vi "Dsc_BoardElecMan.vi"(8 "error in":errorcluster) -> (0 "error out":errorcluster)   [LabVIEW 2014, in "DscBoardDistributeElectrodes.lvlib"]
uses:
  DscBoardDistributeElectrodes.lvlib
  <vilib>/Utility/miscctls.llb/LVRowAndColumnTypeDef.ctl
  DataBase/DataBase.lvlib
  DetectElecrodes/DetectElectros.lvlib
panel:
  out "元素":string
  in  "全部移除":bool
  in  "移除":bool
  in  "采集卡列表":u16(ring) items=["2号数据采集板", "3号数据采集板", "4号数据采集板", "5号数据采集版", "6号数据采集板", "7号数据采集板", "8号数据采集板", "9号数据采集板", "10号数据采集板", "11号数据采集板", "12号数据采集板", "13号数据采集板", "14号数据采集板", "1号数据采集板"]
  in  "已配置 采集卡-检测电极":i32(listbox)
  in  "添加":bool
  in  "电极编号":i32(listbox)
  in  "未配置 采集卡-检测电极":i32(listbox)
  in  "区域":u16(ring)
  in  "退出":bool
  in  "OK":bool
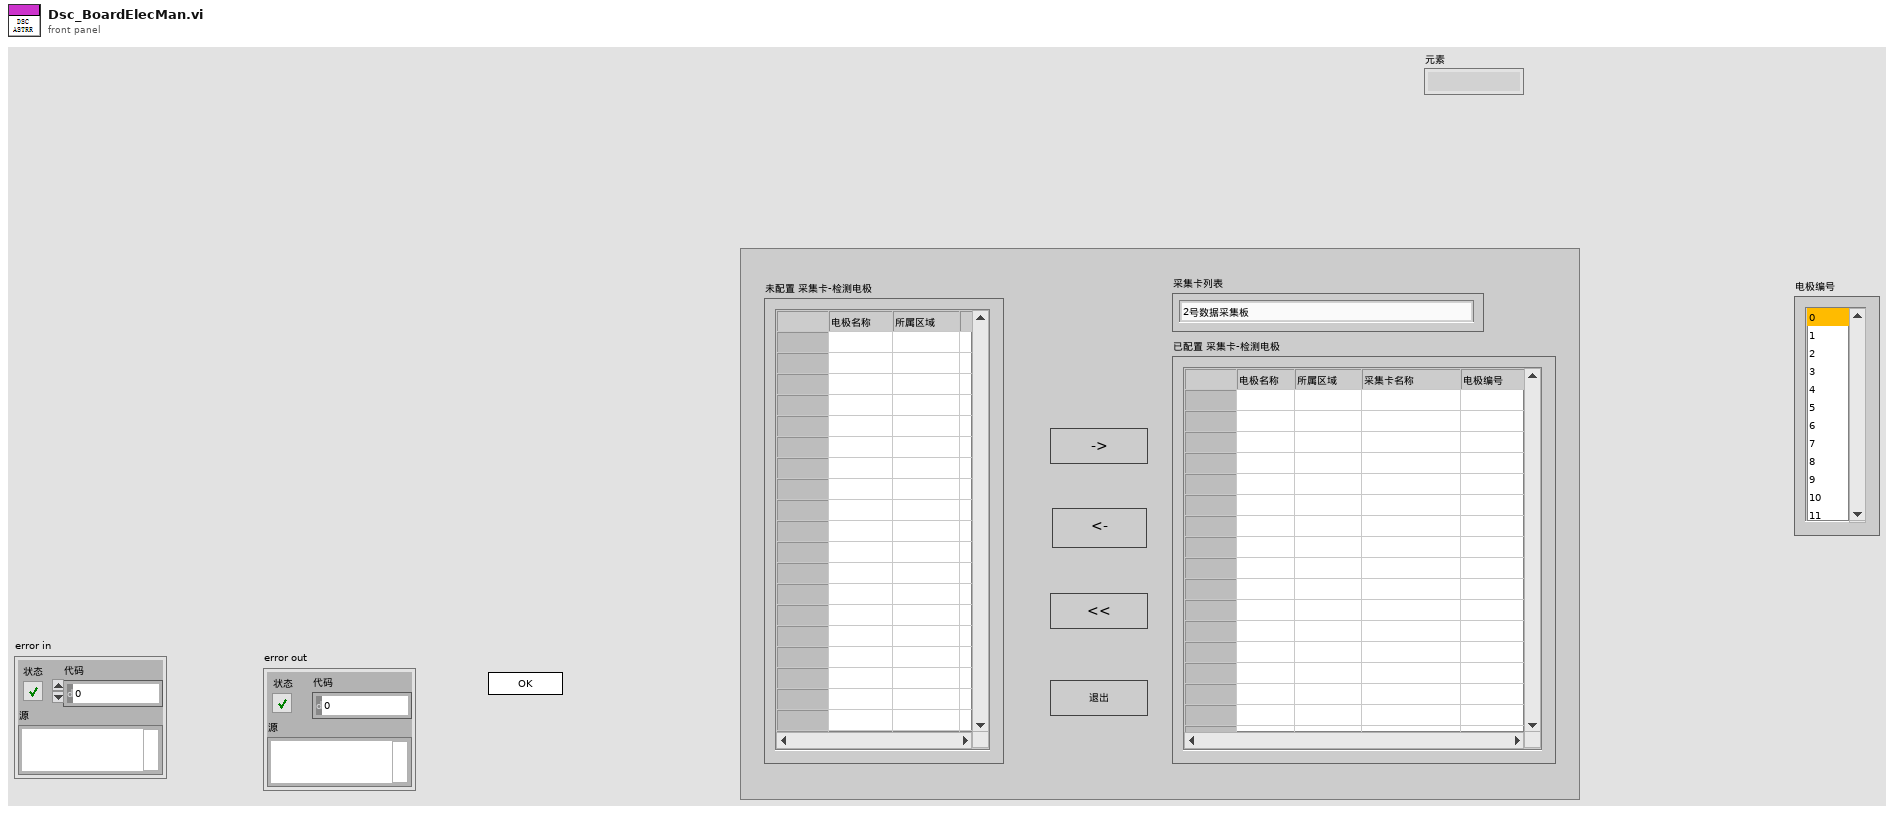
[diagram p1: front panel]
types:
  T1 = enum32{"invalid app kind", "Development System", "Run Time System", "Student Edition", "Embedded LabVIEW", "Evaluation", "Custom"}
  T2 = enum32{"Invalid", "Standard", "Closed", "Hidden", "Minimized", "Maximized"}
  T3 = typedef "LVRowAndColumnTypeDef.ctl" = cluster{"Row":i32, "Column":i32}
  T4 = cluster{"Core":cluster{"Current VI Reference":refnum<vi>, "Close Panel on Exit?":bool}, "Your Boolean data":bool, "Your string data":string, "未配置Dsc行列":T3, "DscInfo":cluster{"DscName":string, "DscAddress":string}, "Dsc":string[][], "Dsc列表":i32, "已配置Dsc行列":T3, "Dsc板名称":string}
  T5 = typedef "LVPoint32TypeDef.ctl" = cluster{"Horizontal":i32, "Vertical":i32}
  T6 = cluster{"Current VI Reference":refnum<vi>, "Close Panel on Exit?":bool}
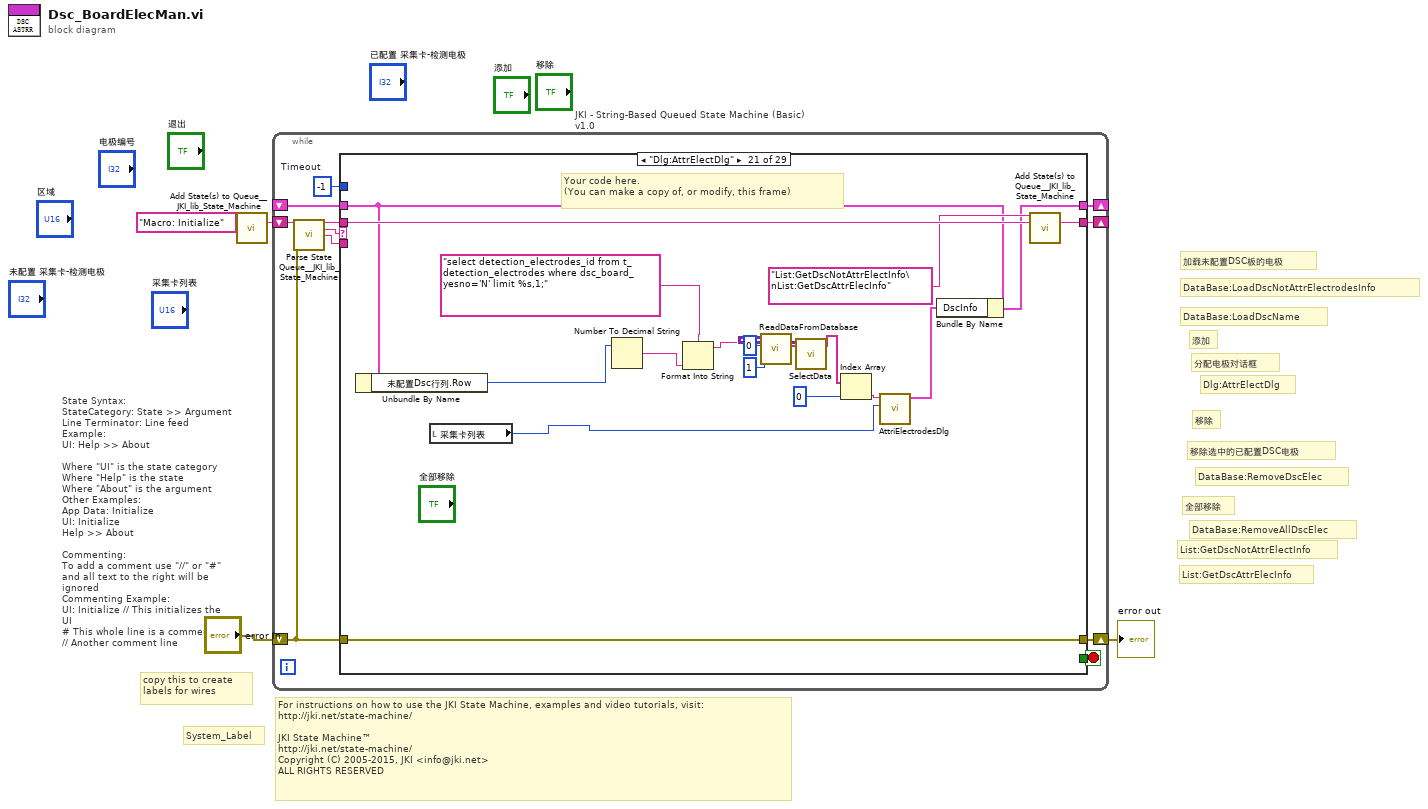
[diagram p0: block diagram]
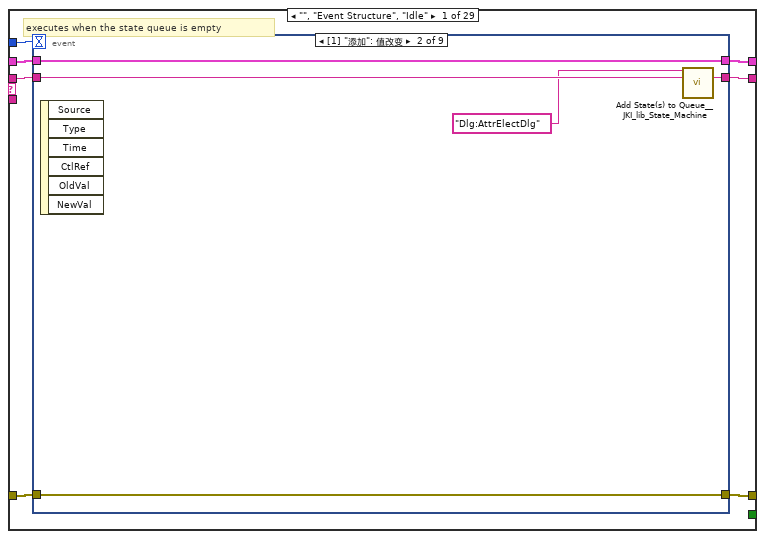
[diagram p2: hidden frame]
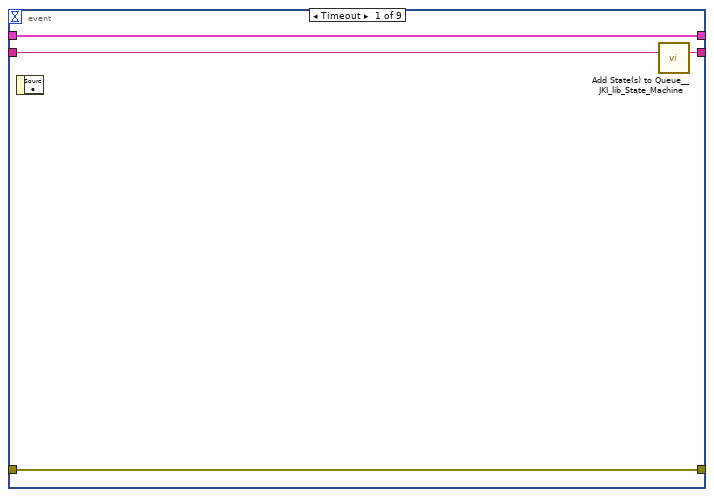
[diagram p3: hidden frame]
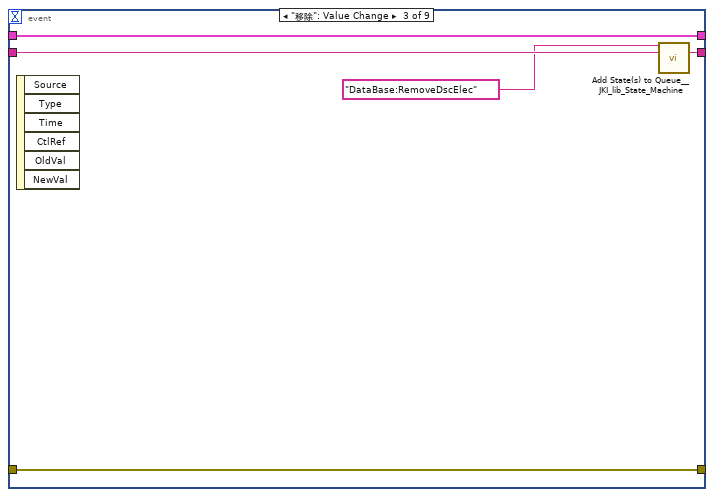
[diagram p4: hidden frame]
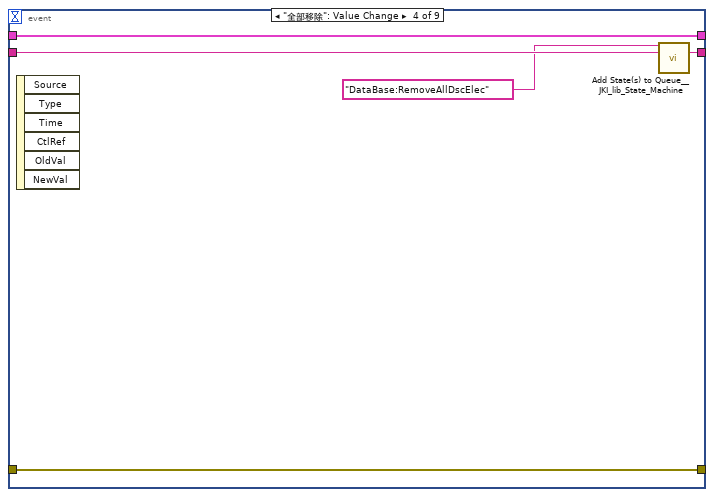
[diagram p5: hidden frame]
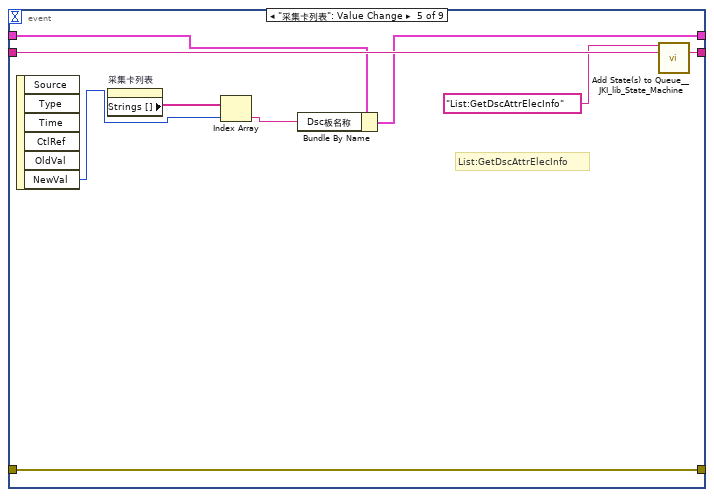
[diagram p6: hidden frame]
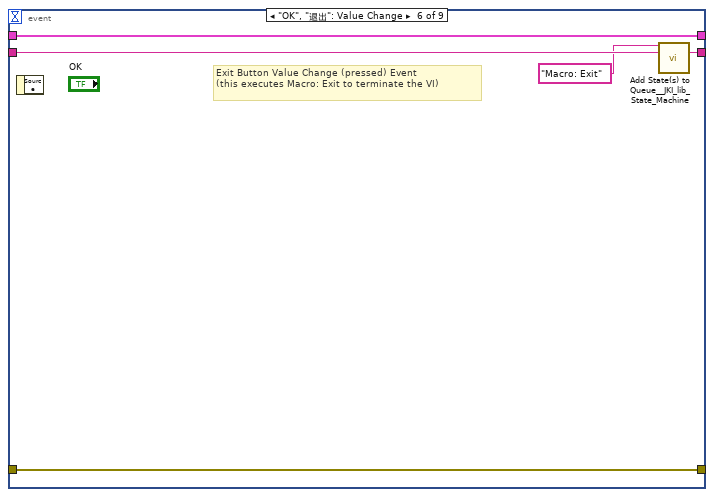
[diagram p7: hidden frame]
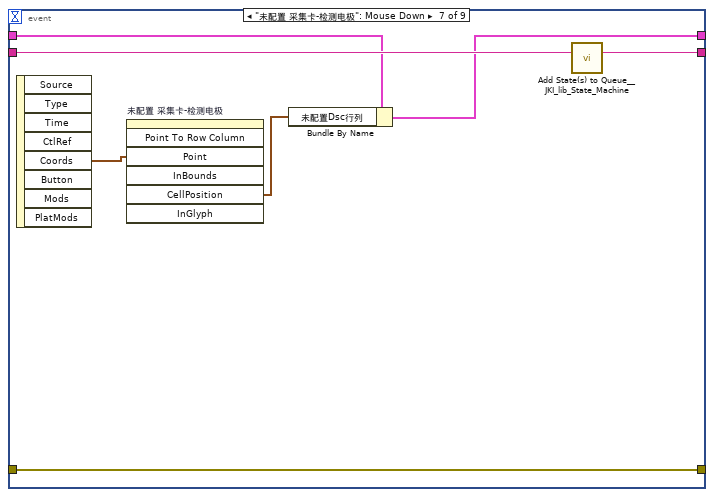
[diagram p8: hidden frame]
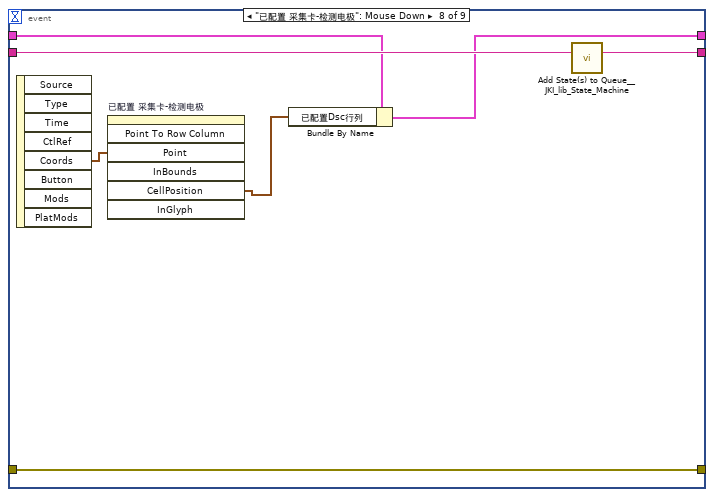
[diagram p9: hidden frame]
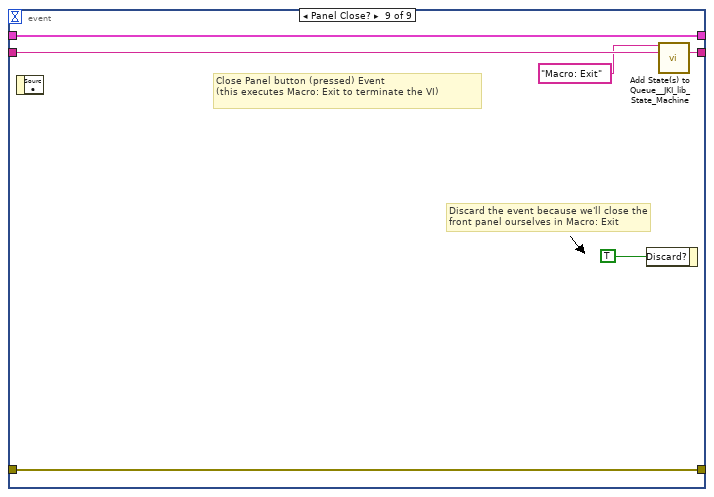
[diagram p10: hidden frame]
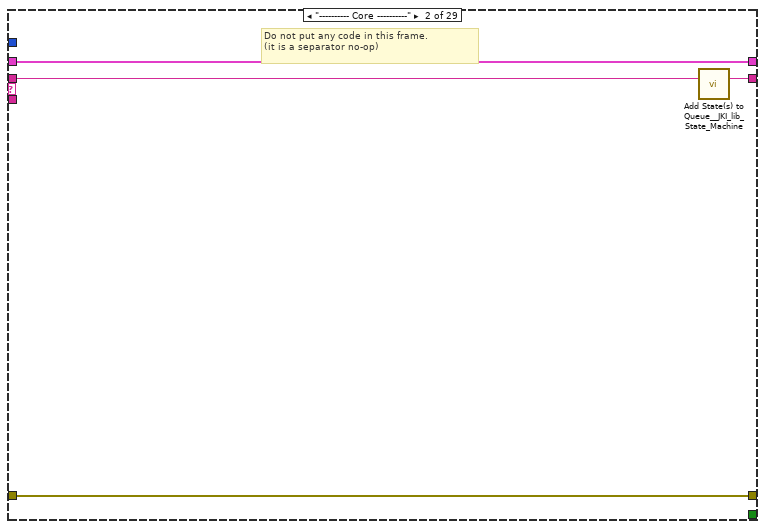
[diagram p11: hidden frame]
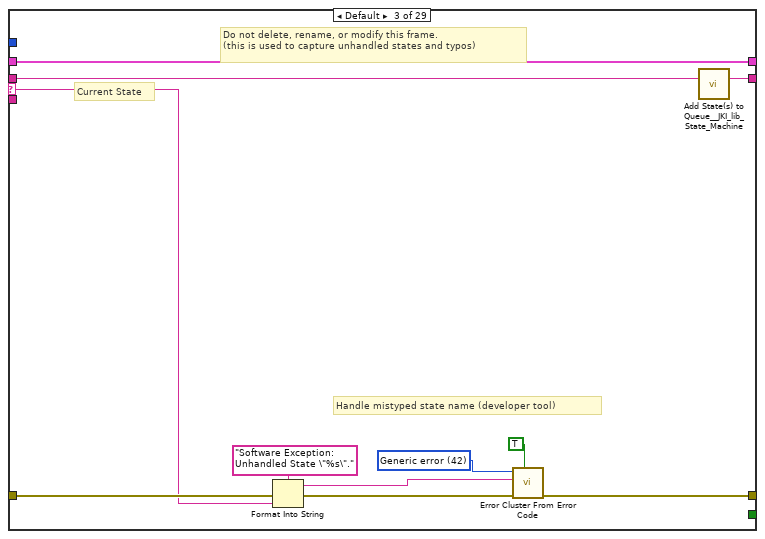
[diagram p12: hidden frame]
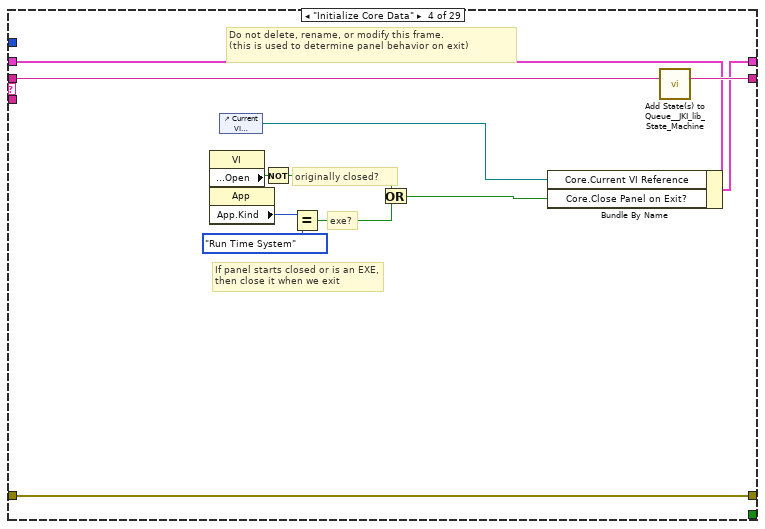
[diagram p13: hidden frame]
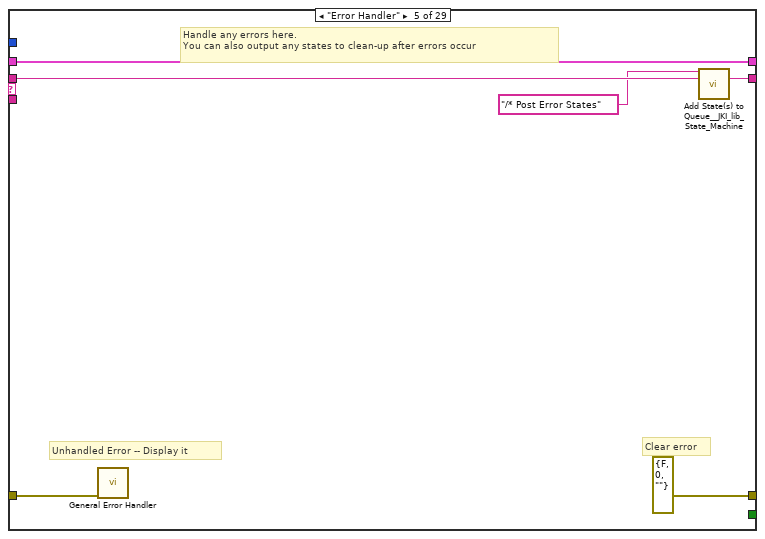
[diagram p14: hidden frame]
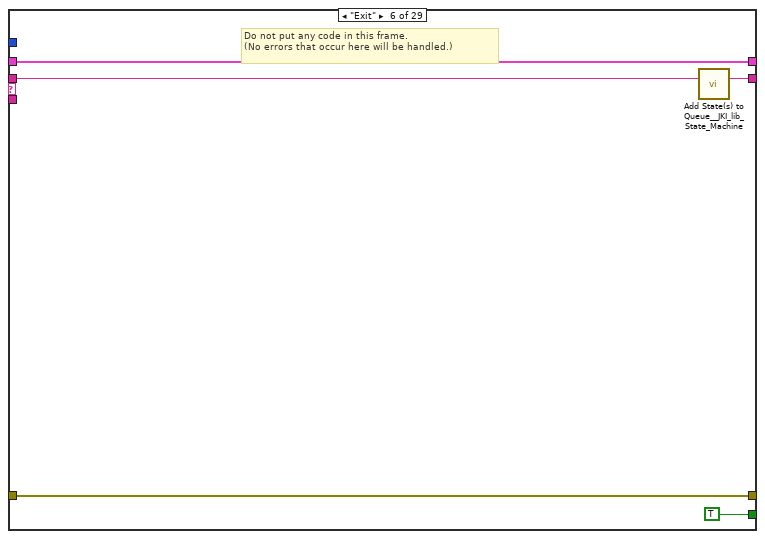
[diagram p15: hidden frame]
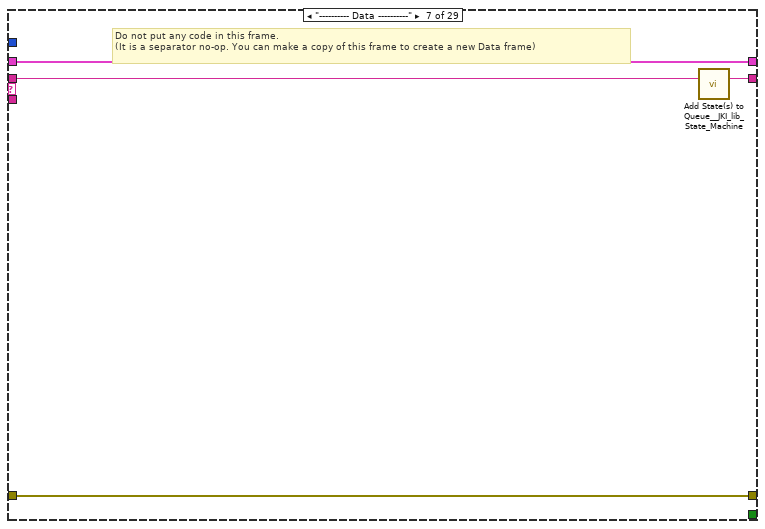
[diagram p16: hidden frame]
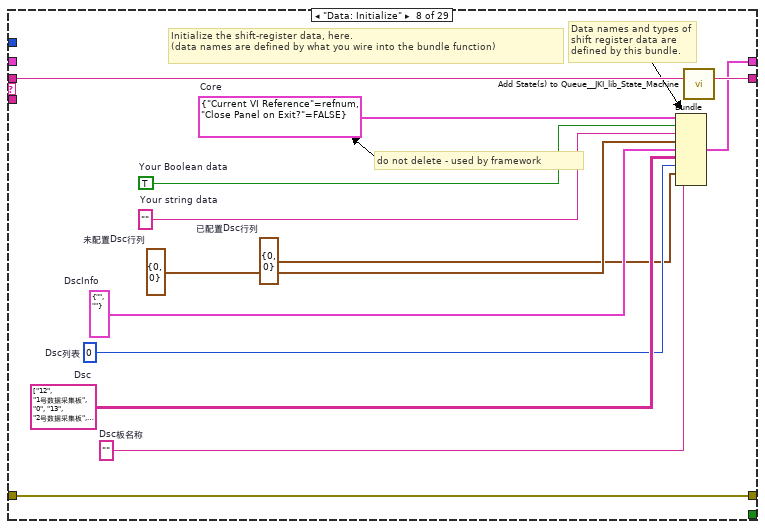
[diagram p17: hidden frame]
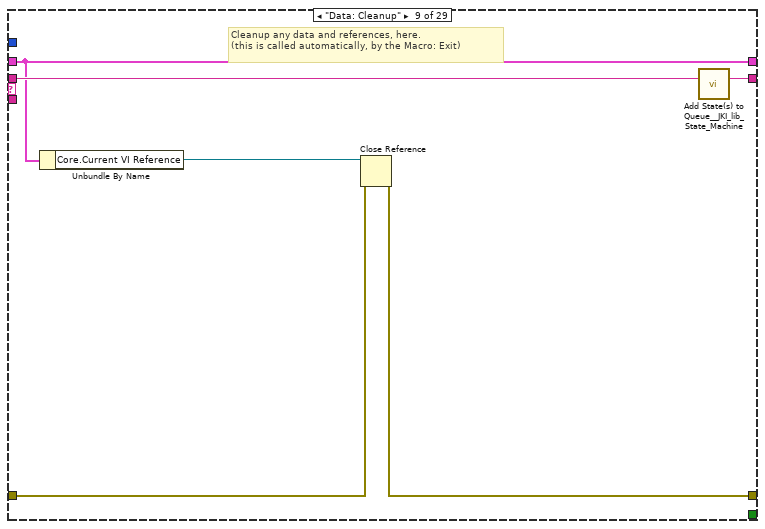
[diagram p18: hidden frame]
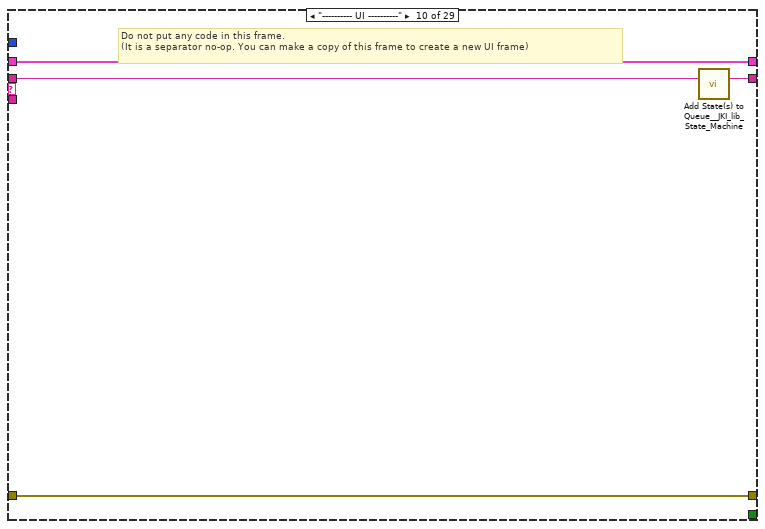
[diagram p19: hidden frame]
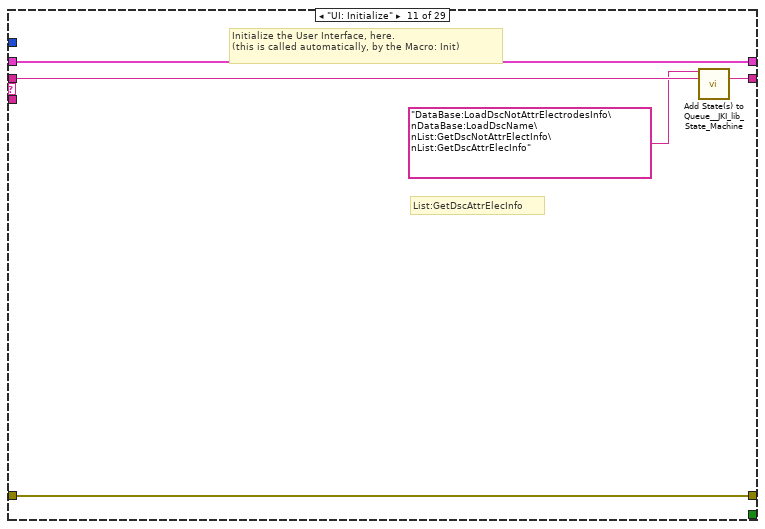
[diagram p20: hidden frame]
diagram:
  # "DataBase:RemoveAllDscElec"
  # "全部移除"
  # "DataBase:RemoveDscElec"
  # "移除选中的已配置DSC电极"
  # "移除"
  # "DataBase:LoadDscName"
  # "List:GetDscAttrElecInfo"
  # "Dlg:AttrElectDlg"
  # "分配电极对话框"
  # "添加"
  # "List:GetDscNotAttrElectInfo"
  # "DataBase:LoadDscNotAttrElectrodesInfo"
  # "加载未配置DSC板的电极"
  # "For instructions on how to use the JKI State Machine, examples and video tutorials, visit:\nhttp://jki.net/state-machine/\n\nJKI State Machine™\nhttp://jki.net/state-machine/\nCopyright (C) 2005-2015, JKI <info@jki.net>\nALL RIGHTS RESERVED"
  # "State Syntax:\nStateCategory: State >> Argument\nLine Terminator: Line feed\nExample:\nUI: Help >> About\n\nWhere \"UI\" is the state category\nWhere \"Help\" is the state\nWhere \"About\" is the argument\nOther Examples:\nApp Data: Initialize\nUI: Initialize\nHelp >> About\n\nCommenting:\nTo add a comment use \"//\" or \"#\" and all text to the right will be ignored\nCommenting Example:\nUI: Initialize // This initializes the UI\n# This whole line is a comment\n// Another comment line"
  # "copy this to create labels for wires"
  # "System_Label"
  n1 = call <vilib>:"Add State(s) to Queue__JKI_lib_State_Machine.vi"("State(s) in (\"\")"="Macro: Initialize") -> ("States Out"=w4:string)  [unwired: 14 in]
  n2 = while "JKI - String-Based Queued State Machine (Basic) v1.0" {
    shift-right: [w8] -> _
    shift-left: _ -> [w7]
    shift-right: [w11] -> w2
    shift-left: "error in" -> [w5]
    shift-right: [w10] -> _
    shift-left: w4 -> [w12]
    stop <- w9 stop-if-true
    w6 = -1  # Timeout
    n3 = call <vilib>:"Parse State Queue__JKI_lib_State_Machine.vi"("State Queue"=w12, "Error In (no error)"=w5) -> ("Remaining States"=w14:string, "Current State"=w15:string, "Arguments"=w13:string)  [unwired: 11 in]
    n4 = case shown="\"Dlg:AttrElectDlg\"" w15 {
      selector: w15 -> [_ _ w80 _ _ _ _ _ _ _ _ _ _ _ _ _ _ _ _ _ _ _ _ _ _ _ _ _ _]
      tunnel: w14 -> [w22 w79 w84 w102 w108 w113 w117 w130 w136 w140 w145 w151 w162 w188 w193 w203 w207 w211 w215 w219 w237 w241 w250 w273 w281 w297 w317 w329 w338]
      tunnel: w13 -> [_ _ _ _ _ _ _ _ _ _ _ w146 w156 _ _ _ _ _ _ _ _ _ _ _ _ _ _ _ _]
      tunnel: w7 -> [w20 w76 w82 w93 w105 w111 w114 _ w131 w137 w143 w149 w158 w185 w190 w200 w204 w208 w212 w216 w221 w238 w247 w270 w278 w294 w314 w320 w335]
      tunnel: [w19 w77 w86 w99 errorcluster {"status"=FALSE, "code"=0, "source"=""} ("error out") w110 w115 w127 w132 w138 w142 w147 w159 w186 w191 w201 w205 w209 w213 w217 w235 w239 w248 w271 w279 w295 w315 w327 w336] -> w11
      tunnel: w5 -> [w18 w77 w85 w99 w104 w110 w115 w127 w133 w138 w142 w148 w160 w186 w191 w201 w205 w209 w213 w217 w235 w239 w248 w271 w279 w295 w315 w327 w336]
      tunnel: [w21 w78 w83 w101 w107 w112 w116 w129 w135 w139 w144 w150 w161 w187 w192 w202 w206 w210 w214 w218 w236 w240 w249 w272 w280 w296 w316 w328 w337] -> w10
      tunnel: [_ _ _ _ _ TRUE _ _ _ _ _ _ _ _ _ _ _ _ _ _ _ _ _ _ _ _ _ _ _] -> w9
      tunnel: [w17 w76 w82 w100 w105 w111 w114 w128 w131 w137 w143 w149 w158 w185 w190 w200 w204 w208 w212 w216 w222 w238 w247 w270 w278 w294 w314 w319 w335] -> w8
      tunnel: w6 -> [w16 _ _ _ _ _ _ _ _ _ _ _ _ _ _ _ _ _ _ _ _ _ _ _ _ _ _ _ _]
      frame "", "Event Structure", "Idle" {
        # "executes when the state queue is empty"
        n5 = event shown="[1] \"添加\": 值改变" {
          selector: _ -> [_ _ _ _ _ _ _ _ _]
          dyn-events: _ -> [_ _ _ _ _ _ _ _ _]
          timeout: w16 -> [_ _ _ _ _ _ _ _ _]
          tunnel: w22 -> [w26 w31 w36 w41 w50 w55 w61 w68 w75]
          tunnel: [w25 w30 w35 w40 w49 w54 w62 w69 w74] -> w21
          tunnel: w20 -> [w23 w28 w33 w38 w44 w52 w57 w66 w72]
          tunnel: [w24 w29 w34 w39 w48 w53 w60 w67 w73] -> w19
          tunnel: w18 -> [w24 w29 w34 w39 w48 w53 w60 w67 w73]
          tunnel: [w23 w28 w33 w38 w42 w52 w56 w65 w72] -> w17
          event Timeout {
            n6 = event-data() -> ()  [unwired: 1 in, 1 out]
            n7 = call <vilib>:"Add State(s) to Queue__JKI_lib_State_Machine.vi"("State(s) in (\"\")"=w26) -> ("States Out"=w25:string)  [unwired: 14 in]
          }
          event "添加": Value Change {
            n8 = event-data() -> ()  [unwired: 1 in, 6 out]
            n9 = call <vilib>:"Add State(s) to Queue__JKI_lib_State_Machine.vi"("State(s) in Front (\"\")"="Dlg:AttrElectDlg", "State(s) in (\"\")"=w31) -> ("States Out"=w30:string)  [unwired: 13 in]
          }
          event "移除": Value Change {
            n10 = event-data() -> ()  [unwired: 1 in, 6 out]
            n11 = call <vilib>:"Add State(s) to Queue__JKI_lib_State_Machine.vi"("State(s) in Front (\"\")"="DataBase:RemoveDscElec", "State(s) in (\"\")"=w36) -> ("States Out"=w35:string)  [unwired: 13 in]
          }
          event "全部移除": Value Change {
            n12 = event-data() -> ()  [unwired: 1 in, 6 out]
            n13 = call <vilib>:"Add State(s) to Queue__JKI_lib_State_Machine.vi"("State(s) in Front (\"\")"="DataBase:RemoveAllDscElec", "State(s) in (\"\")"=w41) -> ("States Out"=w40:string)  [unwired: 13 in]
          }
          event "采集卡列表": Value Change {
            # "List:GetDscAttrElecInfo"
            n14 = event-data() -> ("NewVal"=w45:u16)  [unwired: 1 in, 5 out]
            n15 = property on="采集卡列表" class="Ring (严格)"() -> ("Strings []"=w46:string[])  [unwired: 2 in, 2 out]
            n16 = Index Array(array=w46, index=w45) -> (element=w43:string)
            n17 = Bundle By Name(cluster=w44, "Dsc板名称"=w43) -> (w42:T4)
            n18 = call <vilib>:"Add State(s) to Queue__JKI_lib_State_Machine.vi"("State(s) in Front (\"\")"="List:GetDscAttrElecInfo", "State(s) in (\"\")"=w50) -> ("States Out"=w49:string)  [unwired: 13 in]
          }
          event "OK", "退出": Value Change {
            # "Exit Button Value Change (pressed) Event\n(this executes Macro: Exit to terminate the VI)"
            n19 = event-data() -> ()  [unwired: 1 in, 1 out]
            n20 = call <vilib>:"Add State(s) to Queue__JKI_lib_State_Machine.vi"("State(s) in Front (\"\")"="Macro: Exit", "State(s) in (\"\")"=w55) -> ("States Out"=w54:string)  [unwired: 13 in]
          }
          event "未配置 采集卡-检测电极": Mouse Down {
            n21 = event-data() -> ("Coords"=w59:T5)  [unwired: 1 in, 7 out]
            n22 = invoke on="未配置 采集卡-检测电极" class="MCListbox (严格)" method="Point To Row Column"("Point"=w59) -> ("CellPosition"=w58:T3)  [unwired: 6 in, 6 out]
            n23 = Bundle By Name(cluster=w57, "未配置Dsc行列"=w58) -> (w56:T4)
            n24 = call <vilib>:"Add State(s) to Queue__JKI_lib_State_Machine.vi"("State(s) in (\"\")"=w61) -> ("States Out"=w62:string)  [unwired: 14 in]
          }
          event "已配置 采集卡-检测电极": Mouse Down {
            n25 = event-data() -> ("Coords"=w64:T5)  [unwired: 1 in, 7 out]
            n26 = invoke on="已配置 采集卡-检测电极" class="MCListbox (严格)" method="Point To Row Column"("Point"=w64) -> ("CellPosition"=w63:T3)  [unwired: 6 in, 6 out]
            n27 = Bundle By Name(cluster=w66, "已配置Dsc行列"=w63) -> (w65:T4)
            n28 = call <vilib>:"Add State(s) to Queue__JKI_lib_State_Machine.vi"("State(s) in (\"\")"=w68) -> ("States Out"=w69:string)  [unwired: 14 in]
          }
          event Panel Close? {
            # "Discard the event because we'll close the front panel ourselves in Macro: Exit"
            # "Close Panel button (pressed) Event\n(this executes Macro: Exit to terminate the VI)"
            n29 = event-data() -> ()  [unwired: 1 in, 1 out]
            n30 = event-data("Discard?"=TRUE) -> ()  [unwired: 1 in, 1 out]
            n31 = call <vilib>:"Add State(s) to Queue__JKI_lib_State_Machine.vi"("State(s) in Front (\"\")"="Macro: Exit", "State(s) in (\"\")"=w75) -> ("States Out"=w74:string)  [unwired: 13 in]
          }
        }
      }
      frame "---------- Core ----------" {
        # "Do not put any code in this frame.\n(it is a separator no-op)"
        n32 = call <vilib>:"Add State(s) to Queue__JKI_lib_State_Machine.vi"("State(s) in (\"\")"=w79) -> ("States Out"=w78:string)  [unwired: 14 in]
      }
      frame Default {
        w89 = 42 items=["No error", "Argument error", "Memory is full", "Out of zone", "End of file", "File already open", "Generic file I/O error", "File not found", "File permission error", "Disk is full", "Duplicate path", "Too many files open", "System feature not enabled", "Resource file not found", "Cannot add resource", "Resource not found", "Image not found", "Image memory error", "Pen does not exist", "Config type invalid", "Config token not found", "Config parse error", "Config memory error", "Bad external code format", "Bad external code offset", "External code not present", "Null window", "Destroy window error", "Null menu", "Print aborted", "Bad print record", "Print driver error", "Windows error during printing", "Memory error during printing", "Print dialog error", "Generic print error", "Invalid device refnum", "Device not found", "Device parameter error", "Device unit error", "Cannot open device", "Device call aborted", "Generic error", "Cancelled by user", "Object ID too low", "Object ID too high", "Object not in heap", "Unknown heap", "Unknown object (invalid DefProc)", "Unknown object (DefProc not in table)", "Message out of range", "Invalid (null) method", "Unknown message", "Manager call not supported", "Bad address", "Network operation in progress", "Network operation timed out", "Connection is busy", "Network attribute not supported", "Network error", "Address in use", "System out of memory", "Connection aborted", "Connection refused", "Not connected", "Already connected", "Connection closed", "Initialization error (interapplication manager)", "Bad occurrence", "Wait on unbound occurrence handler", "Occurrence queue overflow", "Datalog type conflict", "Unused", "Unrecognized type (interapplication manager)", "Memory corrupt", "Failed to make temporary DLL", "Old CIN version", "Drag socket not found", "Failed to load drop-object", "Failed to register OLE object", "Failed to release OLE object", "Format specifier type mismatch", "Unknown format specifier", "Too few format specifiers", "Too many format specifiers", "Scan failed", "Newer CIN version", "Error converting to variant", "Runtime menu error", "Password tampered", "Variant attribute not found", "Incompatible variant data type", "Event data is not available", "Event Store is not present", "Occurrence is not found", "Event Queue is not created", "Event info is not available", "Refnum passed is NULL", "Error retrieving Class GUID", "Error retrieving CoClass GUID", "Error retrieving TypeLib GUID.", "Bad built application magic bytes.", "Specific driver is different from the specific driver associated with the Logical Name.", "There is no session opened to the class driver.", "Max Error", "MAX - Error with config objects", "MAX - Error loading configuration", "MAX - Group not supported"]
        # "Current State"
        # "Do not delete, rename, or modify this frame.\n(this is used to capture unhandled states and typos)"
        # "Handle mistyped state name (developer tool)"
        n33 = Format Into String(format string="Software Exception: Unhandled State \"%s\"." ("message"), error in=w85, w80) -> (resulting string=w88:string, error out=w87:errorcluster)  [unwired: 1 in]
        n34 = call <vilib>:"Error Cluster From Error Code.vi"("show call chain? (False)"=TRUE, "error in (no error)"=w87, "error message (\"\")"=w88, "error code (0)"=w89) -> ("error out"=w86:errorcluster)  [unwired: 5 in]
        n35 = call <vilib>:"Add State(s) to Queue__JKI_lib_State_Machine.vi"("State(s) in (\"\")"=w84) -> ("States Out"=w83:string)  [unwired: 14 in]
      }
      frame "Initialize Core Data" {
        # "Do not delete, rename, or modify this frame.\n(this is used to determine panel behavior on exit)"
        # "originally closed?"
        # "exe?"
        # "If panel starts closed or is an EXE, then close it when we exit"
        n36 = property class="VI"() -> ("Front Panel.Open"=w98:bool)  [unwired: 2 in, 2 out]
        n37 = property class="App"() -> ("App.Kind"=w97:T1)  [unwired: 2 in, 2 out]
        n38 = control-ref of="Current VI Reference"() -> (w91:refnum<vi>)
        n39 = Not(x=w98) -> (.not. x?=w95:bool)
        n40 = Equal?(x=w97, y=T1."Run Time System" ("Application:Kind")) -> (x = y?=w94:bool)
        n41 = Or(x=w95, y=w94) -> (x .or. y?=w92:bool)
        n42 = Bundle By Name(cluster=w93, "Core.Current VI Reference"=w91, "Core.Close Panel on Exit?"=w92) -> (w100:T4)
        n43 = call <vilib>:"Add State(s) to Queue__JKI_lib_State_Machine.vi"("State(s) in (\"\")"=w102) -> ("States Out"=w101:string)  [unwired: 14 in]
      }
      frame "Error Handler" {
        # "Unhandled Error -- Display it"
        # "Handle any errors here.\nYou can also output any states to clean-up after errors occur"
        # "Clear error"
        n44 = call <vilib>:"General Error Handler.vi"("error in (no error)"=w104) -> ()  [unwired: 10 in, 5 out]
        n45 = call <vilib>:"Add State(s) to Queue__JKI_lib_State_Machine.vi"("State(s) in Front (\"\")"="/* Post Error States", "State(s) in (\"\")"=w108) -> ("States Out"=w107:string)  [unwired: 13 in]
      }
      frame "Exit" {
        # "Do not put any code in this frame.\n(No errors that occur here will be handled.)"
        n46 = call <vilib>:"Add State(s) to Queue__JKI_lib_State_Machine.vi"("State(s) in (\"\")"=w113) -> ("States Out"=w112:string)  [unwired: 14 in]
      }
      frame "---------- Data ----------" {
        # "Do not put any code in this frame.\n(It is a separator no-op. You can make a copy of this frame to create a new Data frame)"
        n47 = call <vilib>:"Add State(s) to Queue__JKI_lib_State_Machine.vi"("State(s) in (\"\")"=w117) -> ("States Out"=w116:string)  [unwired: 14 in]
      }
      frame "Data: Initialize" {
        w118 = ""  # Dsc板名称
        w119 = T3 {"Row"=0, "Column"=0}  # 已配置Dsc行列
        w120 = 0  # Dsc列表
        w121 = string[][] [["12", "1号数据采集板", "0"], ["13", "2号数据采集板", "1"], ["14", "3号数据采集板", "2"], ["15", "4号数据采集板", "3"]]  # Dsc
        w122 = cluster{"DscName":string, "DscAddress":string} {"DscName"="", "DscAddress"=""}  # DscInfo
        w123 = T3 {"Row"=0, "Column"=0}  # 未配置Dsc行列
        w124 = T6 {"Current VI Reference"=refnum, "Close Panel on Exit?"=FALSE}  # Core
        w126 = TRUE  # Your Boolean data
        w125 = ""  # Your string data
        # "do not delete - used by framework"
        # "Data names and types of shift register data are defined by this bundle."
        # "Initialize the shift-register data, here.\n(data names are defined by what you wire into the bundle function)"
        n48 = Bundle("Core"=w124, "Your Boolean data"=w126, "Your string data"=w125, "未配置Dsc行列"=w123, "DscInfo"=w122, "Dsc"=w121, "Dsc列表"=w120, "已配置Dsc行列"=w119, "Dsc板名称"=w118) -> (w128:T4)  [unwired: 1 in]
        n49 = call <vilib>:"Add State(s) to Queue__JKI_lib_State_Machine.vi"("State(s) in (\"\")"=w130) -> ("States Out"=w129:string)  [unwired: 14 in]
      }
      frame "Data: Cleanup" {
        # "Cleanup any data and references, here.\n(this is called automatically, by the Macro: Exit)"
        n50 = Unbundle By Name(w131) -> ("Core.Current VI Reference"=w134:refnum<vi>)
        n51 = Close Reference(reference=w134, error in (no error)=w133) -> (error out=w132:errorcluster)
        n52 = call <vilib>:"Add State(s) to Queue__JKI_lib_State_Machine.vi"("State(s) in (\"\")"=w136) -> ("States Out"=w135:string)  [unwired: 14 in]
      }
      frame "---------- UI ----------" {
        # "Do not put any code in this frame.\n(It is a separator no-op. You can make a copy of this frame to create a new UI frame)"
        n53 = call <vilib>:"Add State(s) to Queue__JKI_lib_State_Machine.vi"("State(s) in (\"\")"=w140) -> ("States Out"=w139:string)  [unwired: 14 in]
      }
      frame "UI: Initialize" {
        # "List:GetDscAttrElecInfo"
        # "Initialize the User Interface, here.\n(this is called automatically, by the Macro: Init)"
        n54 = call <vilib>:"Add State(s) to Queue__JKI_lib_State_Machine.vi"("State(s) in Front (\"\")"="DataBase:LoadDscNotAttrElectrodesInfo\nDataBase:LoadDscName\nList:GetDscNotAttrElectInfo\nList:GetDscAttrElecInfo", "State(s) in (\"\")"=w145) -> ("States Out"=w144:string)  [unwired: 13 in]
      }
      frame "UI: Cursor Set" {
        # "Argument"
        # "Set and Unset Cursor Busy.\n(Usage: \"UI: Cursor Set >> Busy|Idle\")"
        n55 = case shown="\"Idle\", 默认" w146 {
          tunnel: w148 -> [w153 w155]
          tunnel: [w152 w154] -> w147
          frame "Idle", Default {
            n56 = call <vilib>:"Unset Busy.vi"("error in (no error)"=w153) -> ("error out"=w152:errorcluster)  [unwired: 10 in]
          }
          frame "Busy" {
            n57 = call <vilib>:"Set Busy.vi"("error in (no error)"=w155) -> ("error out"=w154:errorcluster)  [unwired: 9 in, 1 out]
          }
        }
        n58 = call <vilib>:"Add State(s) to Queue__JKI_lib_State_Machine.vi"("State(s) in (\"\")"=w151) -> ("States Out"=w150:string)  [unwired: 14 in]
      }
      frame "UI: Front Panel State" {
        # "Argument"
        # "Set Front Panel Open or Closed\n(Usage: \"UI: Front Panel State >> Open|Close\")"
        n59 = Unbundle By Name(w158) -> ("Core.Current VI Reference"=w157:refnum<vi>)
        n60 = case shown="\"Open\", 默认" w156 {
          tunnel: w160 -> [w166 w179]
          tunnel: [w168 w180] -> w159
          tunnel: w157 -> [w167 w177]
          frame "Open", Default {
            n61 = property class="VI"(reference=w167, error in=w166) -> (reference out=w164:refnum<vi>, error out=w165:errorcluster, "Front Panel.Open"=w163:bool)
            n62 = case shown="假" w163 {
              tunnel: [w171 w174] -> w168
              tunnel: w165 -> [w170 w174]
              tunnel: w164 -> [w169 _]
              frame False {
                n63 = invoke class="VI" method="FP.Open"(reference=w169, error in=w170, "Activate"=TRUE, "State"=T2."Standard") -> (error out=w171:errorcluster)  [unwired: 1 in, 4 out]
              }
              frame True {
              }
            }
          }
          frame "Close" {
            n64 = property class="VI"(reference=w177, error in=w179) -> (reference out=w176:refnum<vi>, error out=w178:errorcluster, "Front Panel.Open"=w175:bool)
            n65 = case shown="真" w175 {
              tunnel: [w181 w184] -> w180
              tunnel: w178 -> [w181 w183]
              tunnel: w176 -> [_ w182]
              frame False {
              }
              frame True {
                n66 = invoke class="VI" method="FP.Close"(reference=w182, error in=w183) -> (error out=w184:errorcluster)  [unwired: 1 in, 2 out]
              }
            }
          }
        }
        n67 = call <vilib>:"Add State(s) to Queue__JKI_lib_State_Machine.vi"("State(s) in (\"\")"=w162) -> ("States Out"=w161:string)  [unwired: 14 in]
      }
      frame "---------- Macro ----------" {
        # "Do not put any code in this frame.\n(It is a separator no-op. You can make a copy of this frame to create a new Macro frame)"
        n68 = call <vilib>:"Add State(s) to Queue__JKI_lib_State_Machine.vi"("State(s) in (\"\")"=w188) -> ("States Out"=w187:string)  [unwired: 14 in]
      }
      frame "Macro: Initialize" {
        w189 = "Data: Initialize\nInitialize Core Data\nUI: Initialize\nUI: Front Panel State >> Open"  # Data: Initialize Initialize Core Data UI: Initialize UI: Front Panel State >> Open
        # "Initialization Macro\n(This is called once, when the VI starts)"
        n69 = call <vilib>:"Add State(s) to Queue__JKI_lib_State_Machine.vi"("State(s) in Front (\"\")"=w189, "State(s) in (\"\")"=w193) -> ("States Out"=w192:string)  [unwired: 13 in]
      }
      frame "Macro: Exit" {
        # "Exit Macro\n(This is called once, when the VI exits)"
        n70 = Unbundle By Name(w200) -> ("Core.Close Panel on Exit?"=w199:bool)
        n71 = Select(t="UI: Front Panel State >> Close", s=w199, f="") -> (s? t:f=w196:string)
        n72 = call <vilib>:"Add State(s) to Queue__JKI_lib_State_Machine.vi"("State(s) in (\"\")"=w196, "State(s) at Back (\"\")"="Data: Cleanup\nExit") -> ("States Out"=w194:string)  [unwired: 13 in]
        n73 = call <vilib>:"Add State(s) to Queue__JKI_lib_State_Machine.vi"("State(s) in Front (\"\")"=w194, "State(s) in (\"\")"=w203) -> ("States Out"=w202:string)  [unwired: 13 in]
      }
      frame "---------- New Category ----------" {
        # "Template Separator\n(You can make a copy of, or modify, this frame)"
        n74 = call <vilib>:"Add State(s) to Queue__JKI_lib_State_Machine.vi"("State(s) in (\"\")"=w207) -> ("States Out"=w206:string)  [unwired: 14 in]
      }
      frame "New Category: 1" {
        # "Your code here.\n(You can make a copy of, or modify, this frame)"
        n75 = call <vilib>:"Add State(s) to Queue__JKI_lib_State_Machine.vi"("State(s) in (\"\")"=w211) -> ("States Out"=w210:string)  [unwired: 14 in]
      }
      frame "New Category: 2" {
        # "Your code here.\n(You can make a copy of, or modify, this frame)"
        n76 = call <vilib>:"Add State(s) to Queue__JKI_lib_State_Machine.vi"("State(s) in (\"\")"=w215) -> ("States Out"=w214:string)  [unwired: 14 in]
      }
      frame "----------Dlg--------" {
        # "Your code here.\n(You can make a copy of, or modify, this frame)"
        n77 = call <vilib>:"Add State(s) to Queue__JKI_lib_State_Machine.vi"("State(s) in (\"\")"=w219) -> ("States Out"=w218:string)  [unwired: 14 in]
      }
      frame "Dlg:AttrElectDlg" {
        # "Your code here.\n(You can make a copy of, or modify, this frame)"
        n78 = Unbundle By Name(w221) -> ("未配置Dsc行列.Row"=w230:i32)
        n79 = local read "采集卡列表"() -> (w220:u16)
        n80 = Number To Decimal String(number=w230) -> (decimal integer string=w231:string)  [unwired: 1 in]
        n81 = Format Into String(format string="select detection_electrodes_id from t_detection_electrodes where dsc_board_yesno='N' limit %s,1;", w231) -> (resulting string=w228:string)  [unwired: 2 in, 1 out]
        n82 = call "SelectData.vi"("SQL query"=w228) -> ("recordset data"=w234:variant[][])  [unwired: 7 in, 1 out]
        n83 = call "ReadDataFromDatabase.vi"("长度"=1, "index"=0, "recordset data"=w234) -> ("一行记录"=w227:string[])  [unwired: 7 in, 1 out]
        n84 = Index Array(array=w227, index=0) -> (element=w225:string)
        n85 = call "AttriElectrodesDlg.vi"("采集卡名称"=w220, "elecID"=w225) -> ("DscInfo"=w223:cluster{"DscName":string, "DscAddress":string})  [unwired: 9 in]
        n86 = Bundle By Name(cluster=w221, "DscInfo"=w223) -> (w222:T4)
        n87 = call <vilib>:"Add State(s) to Queue__JKI_lib_State_Machine.vi"("State(s) in Front (\"\")"="List:GetDscNotAttrElectInfo\nList:GetDscAttrElecInfo", "State(s) in (\"\")"=w237) -> ("States Out"=w236:string)  [unwired: 13 in]
      }
      frame "----------List---------" {
        # "Your code here.\n(You can make a copy of, or modify, this frame)"
        n88 = call <vilib>:"Add State(s) to Queue__JKI_lib_State_Machine.vi"("State(s) in (\"\")"=w241) -> ("States Out"=w240:string)  [unwired: 14 in]
      }
      frame "List:GetDscNotAttrElectInfo" {
        # "加载为配置DSC板的检测电极"
        # "Your code here.\n(You can make a copy of, or modify, this frame)"
        n89 = call "SelectData.vi"("SQL query"="select detection_electrodes_id,detection_electrodes_name,area_name from t_detection_electrodes\nwhere dsc_board_yesno='N'; ") -> ("recordset data"=w245:variant[][])  [unwired: 7 in, 1 out]
        n90 = call "ReadDataFromDatabase.vi"("长度"=3, "index"=1, "recordset data"=w245) -> ("所有记录"=w242:string[][])  [unwired: 7 in, 1 out]
        n91 = property on="未配置 采集卡-检测电极" class="MCListbox (严格)"("ItemNames"=w242) -> ()  [unwired: 2 in, 2 out]
        n92 = call <vilib>:"Add State(s) to Queue__JKI_lib_State_Machine.vi"("State(s) in (\"\")"=w250) -> ("States Out"=w249:string)  [unwired: 14 in]
      }
      frame "List:GetDscAttrElecInfo" {
        # "Your code here.\n(You can make a copy of, or modify, this frame)"
        n93 = Unbundle By Name(w270) -> ("Dsc板名称"=w251:string)
        n94 = Format Into String(format string="select dsc_board_address from t_dsc_board where dsc_board_name='%s';", w251) -> (resulting string=w259:string, error out=w261:errorcluster)  [unwired: 2 in]
        n95 = Build Array(w251) -> (w254:string[])
        n96 = call "SelectData.vi"("SQL query"=w259, "error in"=w261) -> ("recordset data"=w262:variant[][])  [unwired: 6 in, 1 out]
        n97 = call "ReadDataFromDatabase.vi"("长度"=1, "index"=0 ("长度"), "recordset data"=w262) -> ("一行记录"=w257:string[])  [unwired: 7 in, 1 out]
        n98 = Index Array(array=w257, index=0 ("索引")) -> (element=w255:string)
        n99 = Format Into String(format string="select detection_electrodes_name,area_name,dsc_board_electrode_num from \nt_detection_electrodes where dsc_board_yesno='Y' and dsc_board_address='%s' ;", w255) -> (resulting string=w258:string)  [unwired: 2 in, 1 out]
        n100 = call "SelectData.vi"("SQL query"=w258) -> ("recordset data"=w269:variant[][])  [unwired: 7 in, 1 out]
        n101 = call "ReadDataFromDatabase.vi"("长度"=3, "index"=0, "recordset data"=w269) -> ("所有记录"=w266:string[][])  [unwired: 7 in, 1 out]
        n102 = for {
          tunnel: w266 -> [w277] mode=indexing
          tunnel: 2 -> [w274]
          tunnel: [w276] -> w264 mode=indexing
          tunnel: w254 -> [w275]
          n103 = Insert Into Array(array=w277, index=w274, new element=w275) -> (w276:string[])
        }
        n104 = property on="已配置 采集卡-检测电极" class="MCListbox (严格)"("ItemNames"=w264) -> ()  [unwired: 2 in, 2 out]
        n105 = call <vilib>:"Add State(s) to Queue__JKI_lib_State_Machine.vi"("State(s) in (\"\")"=w273) -> ("States Out"=w272:string)  [unwired: 14 in]
      }
      frame "-----------DataBase-----------" {
        # "Your code here.\n(You can make a copy of, or modify, this frame)"
        n106 = call <vilib>:"Add State(s) to Queue__JKI_lib_State_Machine.vi"("State(s) in (\"\")"=w281) -> ("States Out"=w280:string)  [unwired: 14 in]
      }
      frame "DataBase:RemoveAllDscElec" {
        n107 = property on="采集卡列表" class="Ring (严格)"() -> ("Strings []"=w293:string[])  [unwired: 2 in, 2 out]
        n108 = local read "采集卡列表"() -> (w292:u16)
        n109 = Index Array(array=w293, index=w292) -> (element=w283:string)
        n110 = local read "元素"() -> (w282:string)
        n111 = call "SelectData.vi"("SQL query"="select dsc_board_name,dsc_board_address from t_dsc_board;") -> ("recordset data"=w289:variant[][])  [unwired: 7 in, 1 out]
        n112 = Format Into String(format string="update t_detection_electrodes set\ndsc_board_address=null,\ndsc_board_electrode_num=null,\ndsc_board_yesno='N'\nwhere dsc_board_address='%s';", w282) -> (resulting string=w290:string)  [unwired: 2 in, 1 out]
        n113 = call "ReadDataFromDatabase.vi"("长度"=2, "index"=0, "recordset data"=w289) -> ("所有记录"=w285:string[][])  [unwired: 7 in, 1 out]
        n114 = for {
          tunnel: w285 -> [w298] mode=indexing
          tunnel: w283 -> [w300]
          n115 = Index Array(array=w298, index=0 ("索引")) -> (element=w301:string)
          n116 = Equal?(x=w301, y=w300) -> (x = y?=w299:bool)
          n117 = case shown="真" w299 {
            tunnel: w298 -> [_ w305]
            frame False {
            }
            frame True {
              n118 = Index Array(array=w305, index=1 ("索引")) -> (element=→"元素":string)
            }
          }
        }
        n119 = call "updateData.vi"("SQL query"=w290) -> ()  [unwired: 10 in, 1 out]
        n120 = call <vilib>:"Add State(s) to Queue__JKI_lib_State_Machine.vi"("State(s) in Front (\"\")"="List:GetDscNotAttrElectInfo\nList:GetDscAttrElecInfo", "State(s) in (\"\")"=w297) -> ("States Out"=w296:string)  [unwired: 13 in]
      }
      frame "DataBase:RemoveDscElec" {
        # "Your code here.\n(You can make a copy of, or modify, this frame)"
        n121 = Unbundle By Name(w314) -> ("已配置Dsc行列.Row"=w312:i32)
        n122 = property on="已配置 采集卡-检测电极" class="MCListbox (严格)"() -> ("ItemNames"=w313:string[][])  [unwired: 2 in, 2 out]
        n123 = Index Array(array=w313, index (row)=w312) -> (element=w311:string[])  [unwired: 1 in]
        n124 = Index Array(array=w311, index=0 ("索引")) -> (element=w308:string)
        n125 = Format Into String(format string="update t_detection_electrodes set\ndsc_board_address=null,\ndsc_board_electrode_num=null,\ndsc_board_yesno='N'\nwhere detection_electrodes_name='%s';", w308) -> (resulting string=w307:string)  [unwired: 2 in, 1 out]
        n126 = call "updateData.vi"("SQL query"=w307) -> ()  [unwired: 10 in, 1 out]
        n127 = call <vilib>:"Add State(s) to Queue__JKI_lib_State_Machine.vi"("State(s) in Front (\"\")"="List:GetDscNotAttrElectInfo\nList:GetDscAttrElecInfo", "State(s) in (\"\")"=w317) -> ("States Out"=w316:string)  [unwired: 13 in]
      }
      frame "DataBase:LoadDscName" {
        # "Your code here.\n(You can make a copy of, or modify, this frame)"
        n128 = call "SelectData.vi"("SQL query"="select dsc_board_id,dsc_board_name,dsc_board_address\nfrom t_dsc_board;") -> ("recordset data"=w325:variant[][])  [unwired: 7 in, 1 out]
        n129 = call "ReadDataFromDatabase.vi"("长度"=3, "index"=0, "recordset data"=w325) -> ("所有记录"=w318:string[][])  [unwired: 7 in, 1 out]
        n130 = Index Array(array=w318, index (col)=1 ("禁用的索引 (列)")) -> (element=w321:string[])  [unwired: 1 in]
        n131 = Bundle By Name(cluster=w320, "Dsc"=w318) -> (w319:T4)
        n132 = property on="采集卡列表" class="Ring (严格)"("Strings []"=w321) -> ()  [unwired: 2 in, 2 out]
        n133 = call <vilib>:"Add State(s) to Queue__JKI_lib_State_Machine.vi"("State(s) in (\"\")"=w329) -> ("States Out"=w328:string)  [unwired: 14 in]
      }
      frame "DataBase:LoadDscNotAttrElectrodesInfo" {
        # "Your code here.\n(You can make a copy of, or modify, this frame)"
        n134 = call "SelectData.vi"("SQL query"="select detection_electrodes_id,detection_electrodes_name,area_name from t_detection_electrodes\nwhere dsc_board_yesno='N'; ") -> ("recordset data"=w333:variant[][])  [unwired: 7 in, 1 out]
        n135 = call "ReadDataFromDatabase.vi"("长度"=3, "index"=1, "recordset data"=w333) -> ("所有记录"=w330:string[][])  [unwired: 7 in, 1 out]
        n136 = property on="未配置 采集卡-检测电极" class="MCListbox (严格)"("ItemNames"=w330) -> ()  [unwired: 2 in, 2 out]
        n137 = call <vilib>:"Add State(s) to Queue__JKI_lib_State_Machine.vi"("State(s) in (\"\")"=w338) -> ("States Out"=w337:string)  [unwired: 14 in]
      }
    }
  }
  "error out" <- w2
